vi "ProcessData.vi"(8 "error in (no error)":errorcluster, 9 "State":T2, 10 "Analog Data":T3, 11 "TwoAFCeye in":refnum<class "TwoAFCeye.lvclass">) -> (0 "error out":errorcluster, 1 "Fixated":bool, 2 "Trigger":T1=enum."Broke Fixation", 3 "TwoAFCeye out":refnum<class "TwoAFCeye.lvclass">)   [LabVIEW 2010, in "TwoAFCeye.lvclass"]
uses:
  TwoAFCeye.lvclass
  Core SubVIs/Controls/TYPE - Analog Data.ctl
  Trial Based Experiment.lvsc/State.ctl
  Trial Based Experiment.lvsc/Trigger.ctl
  <vilib>/measure/madcrms.llb/Basic Averaged DC-RMS for 1 Chan.vi
  <vilib>/imath/engines/lvmath2/RunTimeEngine/ErrorHandling/NIMS_Finalize Error.vi
  <vilib>/imath/engines/lvmath2/RunTimeEngine/NodeEndStatement/NIMS_NodeEndStatement_Output.vi
  <instcachedir>/0/NIMS_NodeEndStatement_Output_53EC0D466D134D7ABD903AC30B43404B.lvgen/NIMS_NodeEndStatement_Output_53EC0D466D134D7ABD903AC30B43404B_009.vi
  <vilib>/imath/engines/lvmath2/RunTimeEngine/BuiltInFunctions/sum/NIMS_sum(GV).vi
  <instcachedir>/0/NIMS_sum(GV)_67F5EC36BC034E54A6BEC5B0673C00E5.lvgen/NIMS_sum(GV)_67F5EC36BC034E54A6BEC5B0673C00E5_000.vi
  <vilib>/imath/engines/lvmath2/RunTimeEngine/ArithmeticOperatorToken/NIMS_ArithmeticOperator_multmx(RV,CV)-internal.vi
  <instcachedir>/0/NIMS_ArithmeticOperator_multmx(RV,CV)-internal_40FB8BE34F5D4DB2AA4F480203295D22.lvgen/NIMS_ArithmeticOperator_multmx(RV,CV)-internal_40FB8BE34F5D4DB2AA4F480203295D22_006.vi
  <vilib>/imath/engines/lvmath2/RunTimeEngine/BuiltInFunctions/abs/NIMS_abs(signed).vi
  <instcachedir>/0/NIMS_abs(signed)_C4FCB8E6058B49B797C7C8D53CA5F6EC.lvgen/NIMS_abs(signed)_C4FCB8E6058B49B797C7C8D53CA5F6EC_002.vi
  <vilib>/imathl/engines/lvmath/Functions/Error Handling/Create Error.vi
  Core SubVIs/Core SubVIs.lvlib
  <vilib>/measure/NI_MAPro.lvlib
  Trial Based Experiment.lvsc
  Matlab API/Matlab API.lvlib
panel:
  in  "Adjustment Rate":dbl=0.02
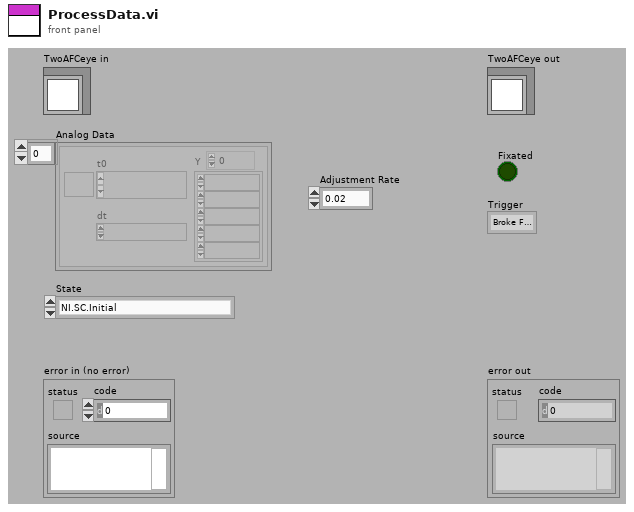
[diagram p1: front panel]
types:
  T1 = typedef "Trial Based Experiment.lvsc/Trigger.ctl" = enum16{"NULL", "Fixated", "Broke Fixation", "Stop", "Correct Response", "Incorrect Response", "Timeout"}
  T2 = typedef "Trial Based Experiment.lvsc/State.ctl" = enum16{"NI.SC.Initial", "NI.SC.History", "NI.SC.ShallowHistory", "NI.SC.Terminal", "Cleanup", "State", "State\\Region\\Pause", "State\\Region\\Response Period", "State\\Region\\Delay Period", "State\\Region\\Hold Fixation", "State\\Region\\Acquire Fixation", "State\\Region\\Abort Trial", "State\\Region\\End Trial", "State\\Region\\Intertrial", "State\\Region\\Start Trial"}
  T3 = typedef "Core SubVIs.lvlib/TYPE - Analog Data.ctl" = waveform(dbl)[]
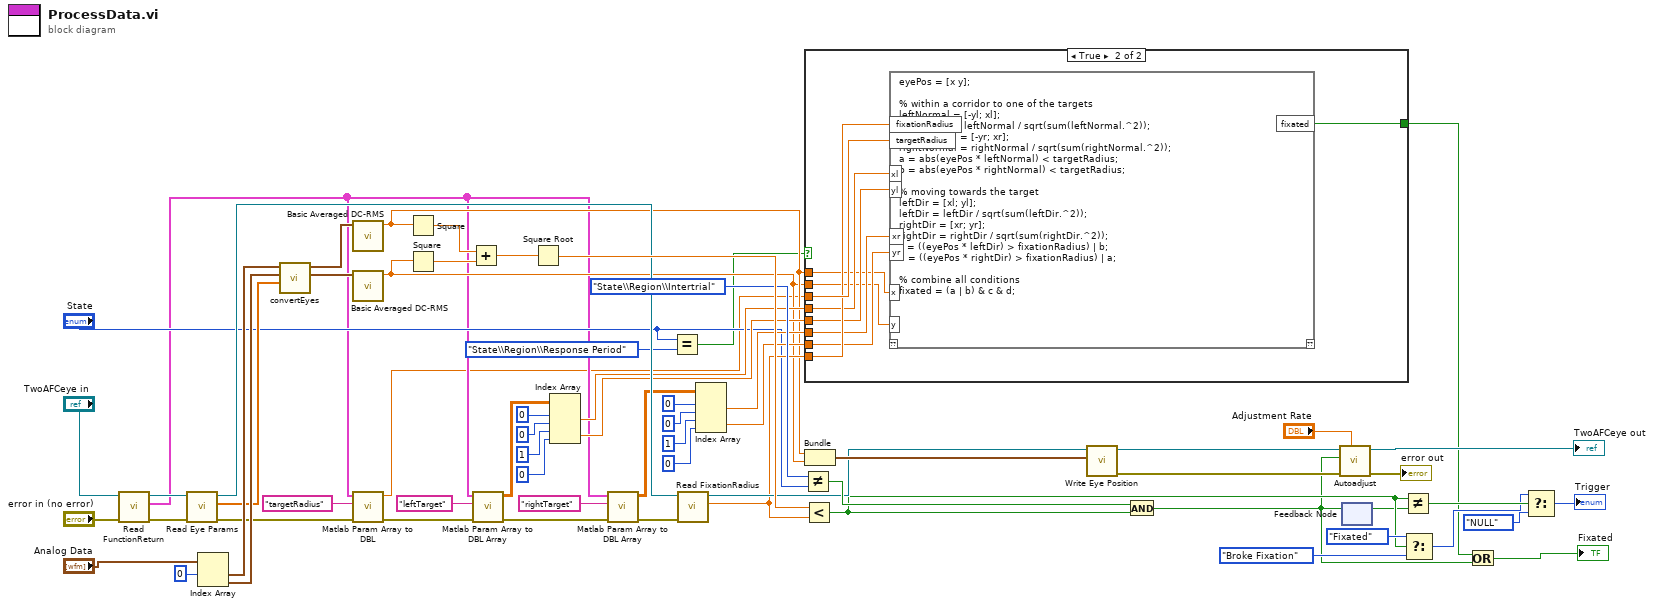
[diagram p0: block diagram]
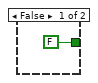
[diagram p2: hidden frame]
diagram:
  n1 = call-dynamic "Read FunctionReturn.vi"("error in (no error)"="error in (no error)", "MatlabExperiment in"="TwoAFCeye in") -> ("error out"=w16:errorcluster, "FunctionReturn"=w6:cluster{"Name":string, "Data":variant}[], "MatlabExperiment out"=w15:refnum<class "TwoAFCeye.lvclass">)  [unwired: 7 in]
  n2 = call-dynamic "Read Eye Params.vi"("error in (no error)"=w16, "TrialBasedExperiment in"=w15) -> ("error out"=w4:errorcluster, "Eye Params"=w40:dbl[], "TrialBasedExperiment out"=w45:refnum<class "TwoAFCeye.lvclass">)  [unwired: 7 in]
  n3 = Index Array(array="Analog Data", index #1=0 ("index")) -> (element #1=w42:waveform(dbl), element #2=w41:waveform(dbl))  [unwired: 1 in]
  n4 = call "convertEyes.vi"("Params"=w40, "Vertical"=w41, "Horizontal"=w42) -> ("Vertical Calibrated"=w59:waveform(dbl), "Horizontal Calibrated"=w60:waveform(dbl))  [unwired: 7 in]
  n5 = call-poly <vilib>:"Basic Averaged DC-RMS.vi"("signal in"=w60) -> ("DC value"=w13:dbl)  [unwired: 7 in, 3 out]
  n6 = call-poly <vilib>:"Basic Averaged DC-RMS.vi"("signal in"=w59) -> ("DC value"=w12:dbl)  [unwired: 7 in, 3 out]
  n7 = call "Matlab Param Array to DBL.vi"("error in (no error)"=w4, "Name"="targetRadius", "Matlab Param Array"=w6) -> ("error out"=w3:errorcluster, "data"=w5:dbl)  [unwired: 7 in]
  n8 = Square(x=w13) -> (x^2=w62:dbl)
  n9 = Square(x=w12) -> (x^2=w63:dbl)
  n10 = Add(x=w62, y=w63) -> (x+y=w64:dbl)
  n11 = call "Matlab Param Array to DBL Array.vi"("error in (no error)"=w3, "Name"="leftTarget", "Matlab Param Array"=w6) -> ("error out"=w2:errorcluster, "data"=w20:dbl[][])  [unwired: 7 in]
  n12 = Square Root(x=w64) -> (sqrt(x)=w65:dbl)
  n13 = Index Array(array=w20, index (row) #1=0 ("index"), index (col) #1=0 ("disabled index (col)"), index (row) #2=1 ("index"), index (col) #2=0 ("disabled index (col)")) -> (element #1=w32:dbl, element #2=w33:dbl)
  n14 = call "Matlab Param Array to DBL Array.vi"("error in (no error)"=w2, "Name"="rightTarget", "Matlab Param Array"=w6) -> ("error out"=w1:errorcluster, "data"=w18:dbl[][])  [unwired: 7 in]
  n15 = Equal?(x="State", y=State."State\\Region\\Response Period") -> (x = y?=w7:bool)
  n16 = call-dynamic "Read FixationRadius.vi"("error in (no error)"=w1, "MatlabExperiment in"=w45) -> ("FixationRadius"=w14:dbl, "MatlabExperiment out"=w44:refnum<class "TwoAFCeye.lvclass">)  [unwired: 7 in, 1 out]
  n17 = Index Array(array=w18, index (row) #1=0 ("index"), index (col) #1=0 ("disabled index (col)"), index (row) #2=1 ("index"), index (col) #2=0 ("disabled index (col)")) -> (element #1=w34:dbl, element #2=w35:dbl)
  n18 = Not Equal?(x=State."State\\Region\\Intertrial", y="State") -> (x != y?=w49:bool)
  n19 = Less?(x=w65, y=w14) -> (x < y?=w38:bool)
  n20 = case shown="True" w7 {
    tunnel: [FALSE w74] -> w36
    tunnel: w5 -> [_ w75]
    tunnel: w32 -> [_ w72]
    tunnel: w33 -> [_ w71]
    tunnel: w34 -> [_ w70]
    tunnel: w35 -> [_ w69]
    tunnel: w14 -> [_ w73]
    tunnel: w13 -> [_ w68]
    tunnel: w12 -> [_ w67]
    frame False {
    }
    frame True {
      n21 = mathscript code="eyePos = [x y];\n\n% within a corridor to one of the targets\nleftNormal = [-yl; xl];\nleftNormal = leftNormal / sqrt(sum(leftNormal.^2));\nrightNormal = [-yr; xr];\nrightNormal = rightNormal / sqrt(sum(rightNormal.^2));\na = abs(eyePos * leftNormal) < targetRadius;\nb = abs(eyePos * rightNormal) < targetRadius;\n\n% moving towards the target\nleftDir = [xl; yl];\nleftDir = leftDir / sqrt(sum(leftDir.^2));\nrightDir = [xr; yr];\nrightDir = rightDir / sqrt(sum(rightDir.^2));\nc = ((eyePos * leftDir) > fixationRadius) | b;\nd = ((eyePos * rightDir) > fixationRadius) | a;\n\n% combine all conditions\nfixated = (a | b) & c & d;"("xl"=w72, "yl"=w71, "xr"=w70, "yr"=w69, "fixationRadius"=w73, "targetRadius"=w75, "x"=w68, "y"=w67) -> ("fixated"=w74:bool)  [unwired: 1 in, 1 out]
    }
  }
  n22 = Bundle("DC value"=w13, "DC value"=w12) -> (w46:cluster{"DC value":dbl, "DC value":dbl})  [unwired: 1 in]
  n23 = call-dynamic "Write Eye Position.vi"("Eye Position"=w46, "TrialBasedExperiment in"=w44) -> ("error out"=w58:errorcluster, "TrialBasedExperiment out"=w56:refnum<class "TwoAFCeye.lvclass">)  [unwired: 8 in]
  n24 = And(x=w49, y=w38) -> (x .and. y?=w10:bool)
  n25 = call-dynamic "Autoadjust.vi"("Adjustment Rate"="Adjustment Rate", "error in (no error)"=w58, "Fixated"=w10, "TrialBasedExperiment in"=w56) -> ("error out"=→"error out":errorcluster, "TrialBasedExperiment out"=→"TwoAFCeye out":refnum<class "TwoAFCeye.lvclass">)  [unwired: 6 in]
  n26 = feedback #1() -> (w37:bool)  [unwired: 1 in]
  n27 = feedback-in #1(w10) -> ()
  n28 = Not Equal?(x=w38, y=w37) -> (x != y?=w55:bool)
  n29 = Select(t=Trigger."Fixated" ("Trigger"), s=w38, f=Trigger."Broke Fixation" ("Trigger")) -> (s? t:f=w52:T1)
  n30 = Or(x=w36, y=w10) -> (x .or. y?=→"Fixated":bool)
  n31 = Select(t=w52, s=w55, f=Trigger."NULL" ("Trigger")) -> (s? t:f=→"Trigger":T1)
